vi "SP Derivative x(t).vi"(2 "dt":dbl=1.0 format="%0.2f", 3 "final condition":dbl format="%0.2f", 4 "initial condition":dbl format="%0.2f", 5 "X":dbl[](array[numeric])) -> (0 "error":i32, 1 "dX/dt":dbl[](array[numeric]))   [LabVIEW 2011]
doc: "Performs a discrete differentiation of the sampled signal <B>X</B>."
uses:
  LabVIEW 2009/resource/lvanlys.dll
panel:
  # "dx(t)/dt"
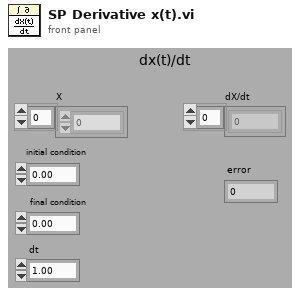
[diagram p1: front panel]
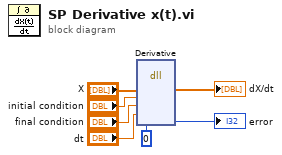
[diagram p0: block diagram]
diagram:
  n1 = dll-call lib="C:/Development/LabVIEW 2009/resource/lvanlys.*" fn="Derivative"("X"="X", "initial condition"="initial condition", "final condition"="final condition", "dt"="dt", "output param"=0) -> ("X"=→"dX/dt":dbl[], "output param"=→"error":i32)  [unwired: 6 in, 3 out]
